vi "数组案例之数字个数计算(上).vi"() -> ()   [LabVIEW 2018]
panel:
  out "数组 2":dbl[](array[numeric])
  out "已排序的数组":dbl[](array[numeric])
  in  "数组":dbl[](array[numeric])
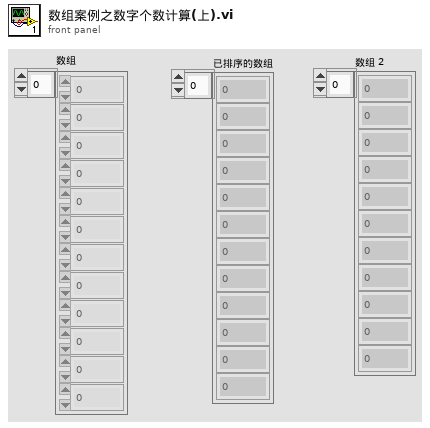
[diagram p1: front panel]
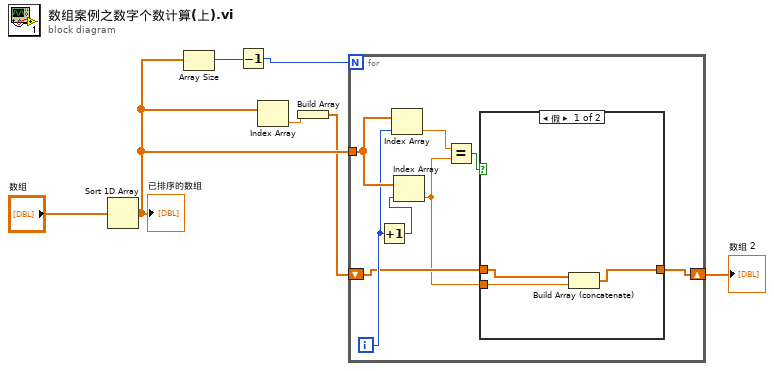
[diagram p0: block diagram]
diagram:
  n1 = Sort 1D Array(array="数组") -> (sorted array=w4:dbl[])
  "已排序的数组" <- w4
  n2 = Array Size(array=w4) -> (size(s)=w6:i32)
  n3 = Decrement(x=w6) -> (x-1=w5:i32)
  n4 = Index Array(array=w4) -> (element=w3:dbl)  [unwired: 1 in]
  n5 = Build Array(w3) -> (w2:dbl[])
  n6 = for {
    N: w5 -> [_]
    tunnel: w4 -> [w15]
    shift-right: [w9] -> w1
    shift-left: w2 -> [w10]
    i -> [w13]
    n7 = Increment(x=w13) -> (x+1=w14:i32)
    n8 = Index Array(array=w15, index=w13) -> (element=w12:dbl)
    n9 = Index Array(array=w15, index=w14) -> (element=w8:dbl)
    n10 = Equal?(x=w12, y=w8) -> (x = y?=w11:bool)
    n11 = case shown="假" w11 {
      tunnel: w10 -> [w18 w19]
      tunnel: [w16 w19] -> w9
      tunnel: w8 -> [w17 _]
      frame False {
        n12 = Build Array (concatenate)(w18, w17) -> (w16:dbl[])
      }
      frame True {
      }
    }
  }
  "数组 2" <- w1
